vi "Save Transport DAT File.vi"(8 "error in (no error)":errorcluster, 10 "Data (Row)":dbl[](array[numeric]), 11 "Control Experiment in":refnum<class "Control Experiment.lvclass">) -> (0 "error out":errorcluster)   [LabVIEW 2016, in "Control Experiment.lvclass"]
uses:
  Control Experiment.lvclass
  Control Experiment.lvclass/Control Experiment.ctl
  <userlib>/LevyLab/LV to ITX/LVtoITX.lvclass
panel:
  out "Control Experiment out":refnum<class "Control Experiment.lvclass">
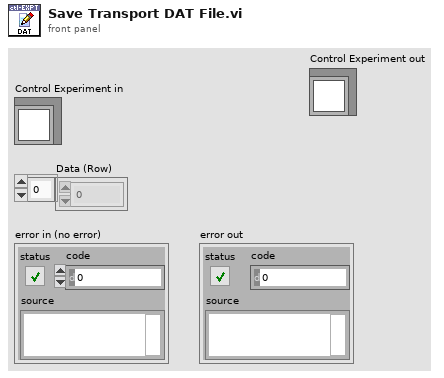
[diagram p1: front panel]
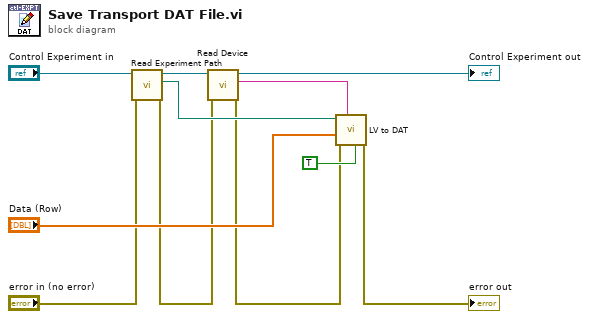
[diagram p0: block diagram]
diagram:
  n1 = call "Read Experiment Path.vi"("error in (no error)"="error in (no error)", "Control Experiment in"="Control Experiment in") -> ("error out"=w3:errorcluster, "Experiment Path"=w8:path, "Control Experiment out"=w6:refnum<class "Control Experiment.lvclass">)  [unwired: 7 in]
  n2 = call "Read Device.vi"("error in (no error)"=w3, "Control Experiment in"=w6) -> ("error out"=w2:errorcluster, "Device"=w9:string, "Control Experiment out"=→"Control Experiment out":refnum<class "Control Experiment.lvclass">)  [unwired: 7 in]
  n3 = call <userlib>:"LV to DAT.vi"("append to file? (new file:F)"=TRUE, "filename"=w9, "error in"=w2, "Data"="Data (Row)", "path"=w8) -> ("error out"=→"error out":errorcluster)  [unwired: 5 in, 1 out]
